vi "PGPASS.ConnectionMgr.vi"(8 "error in (no error)":errorcluster) -> (0 "error out":errorcluster, 3 "Connection":T1)   [LabVIEW 2019, in "PGPASS.lvlib"]
uses:
  PGPASS.lvlib
  PGPASS.Connection Information.ctl
  <vilib>/JDP Science/PostgreSQL Library/Connection/Execute Command (1D string results).vi
  <vilib>/JDP Science/PostgreSQL Library/Connection/Execute Command (Result).vi
  <vilib>/JDP Science/PostgreSQL Library/Result/Get all results as 1D strings array.vi
  <vilib>/JDP Science/PostgreSQL Library/Result/Get Column Headers.vi
  <vilib>/JDP Science/PostgreSQL Library/Result/Clear.vi
  <vilib>/JDP Science/PostgreSQL Library/Connection/PQ Connection.lvclass
panel:
  in  "CANCEL":bool
  out "Status":string
  in  "Validate":bool
  in  "Connections":i32(listbox)
  in  "Exit":bool
  in  "Delete Connection":bool
  in  "Add Connection":bool
  in  "Host":string
  in  "Port":string
  in  "Database":string
  in  "Username":string
  in  "Password":string
  # "PGPASS: Connection Manager"
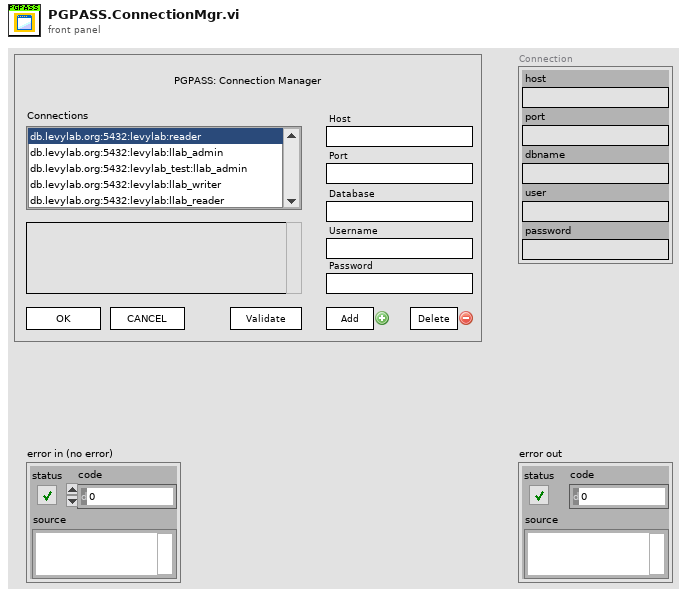
[diagram p1: front panel]
types:
  T1 = typedef "PGPASS.lvlib/PGPASS.Connection Information.ctl" = cluster{"host":string, "port":string, "dbname":string, "user":string, "password":string}
  T2 = enum32{"Invalid", "Standard", "Closed", "Hidden", "Minimized", "Maximized"}
  T3 = enum32{"invalid app kind", "Development System", "Run Time System", "Student Edition", "Embedded LabVIEW", "Evaluation", "Custom"}
  T4 = cluster{"Core":cluster{"Current VI Reference":refnum<vi>, "Close Panel on Exit?":bool}, "All Connections":T1[], "Connection":T1}
  T5 = cluster{"Current VI Reference":refnum<vi>, "Close Panel on Exit?":bool}
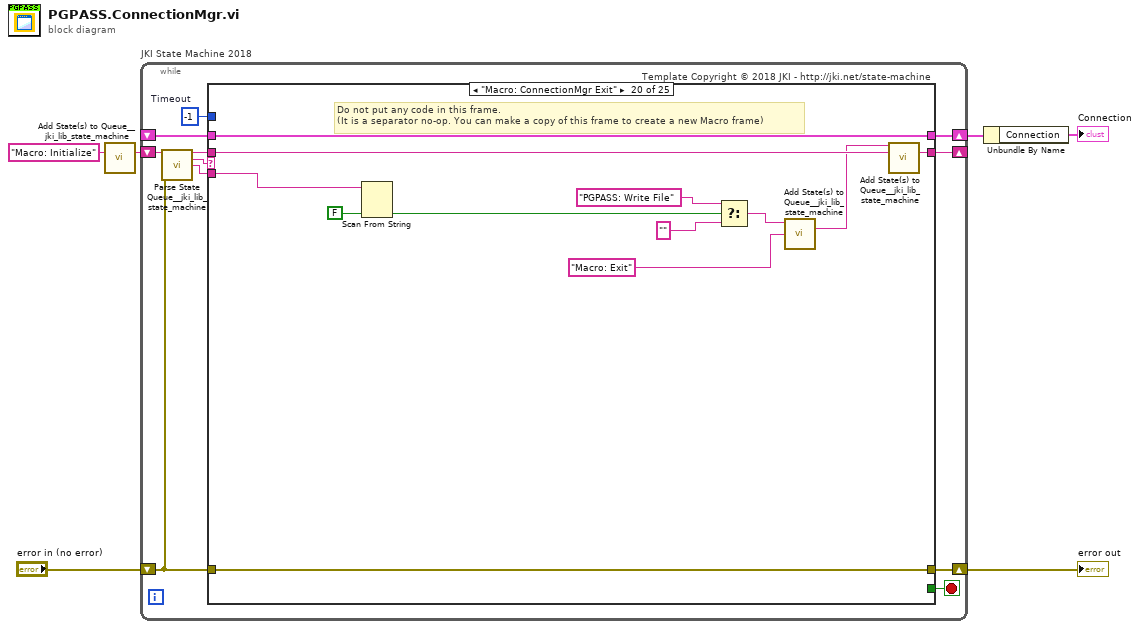
[diagram p0: block diagram]
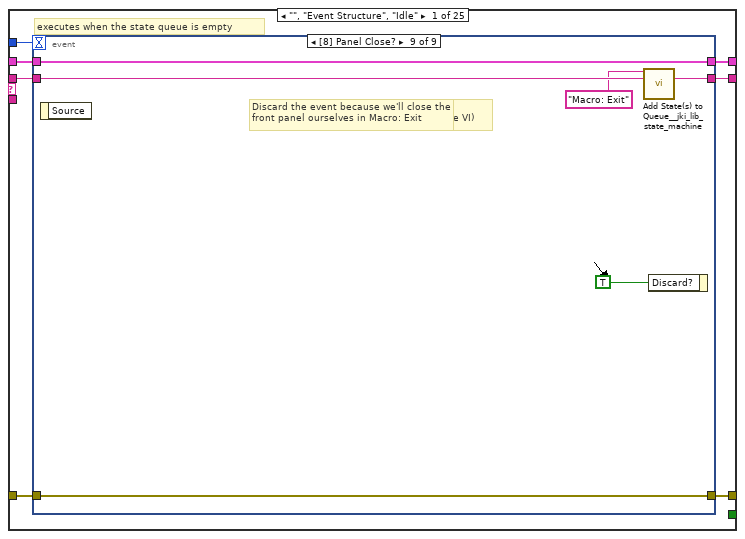
[diagram p2: hidden frame]
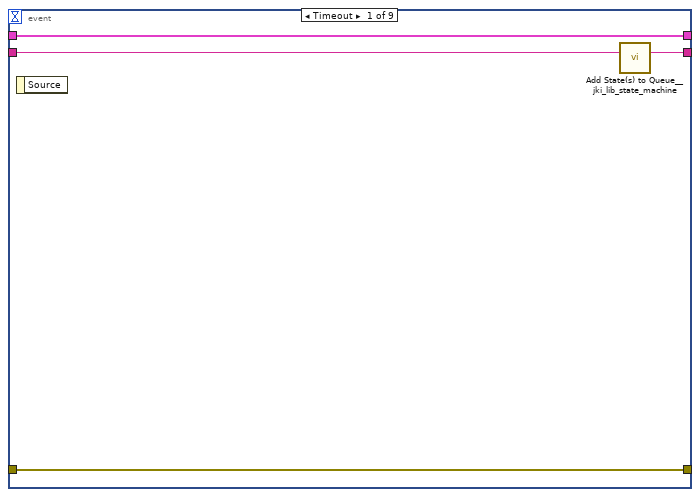
[diagram p3: hidden frame]
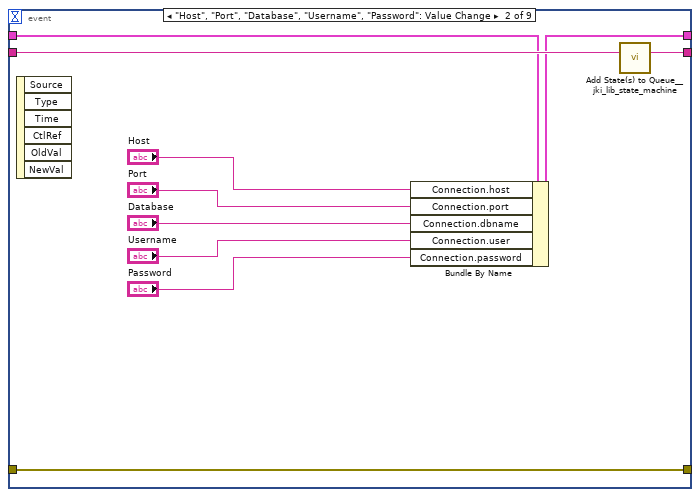
[diagram p4: hidden frame]
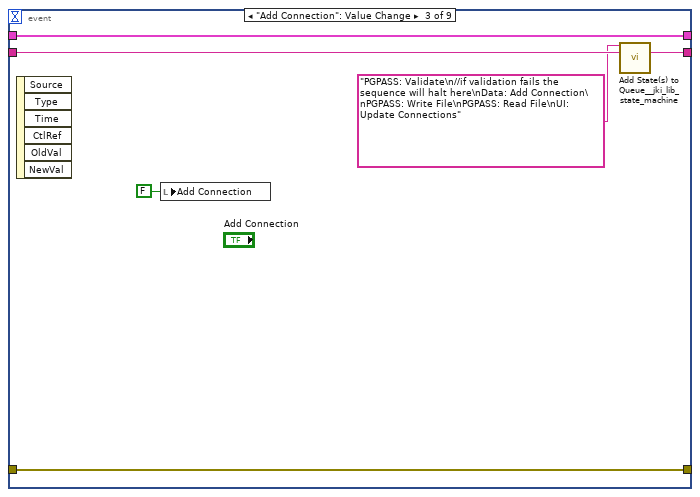
[diagram p5: hidden frame]
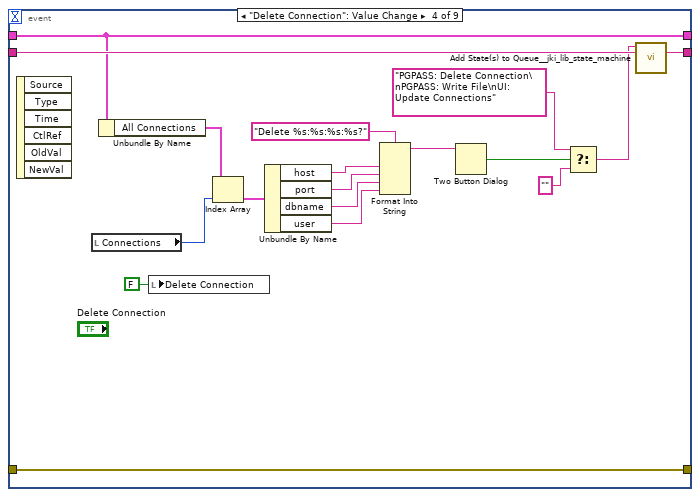
[diagram p6: hidden frame]
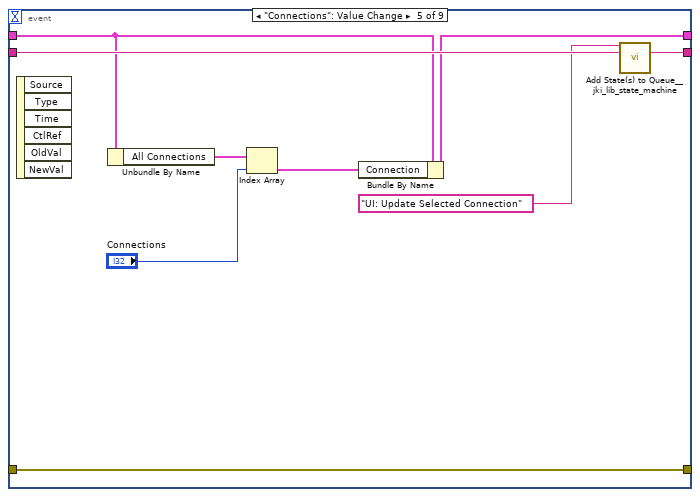
[diagram p7: hidden frame]
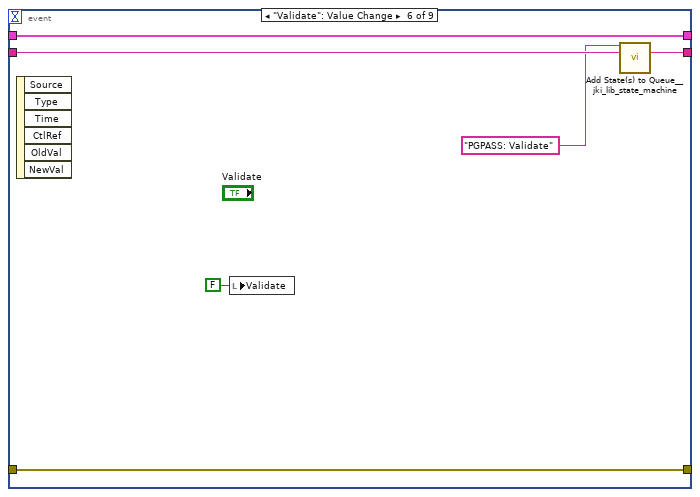
[diagram p8: hidden frame]
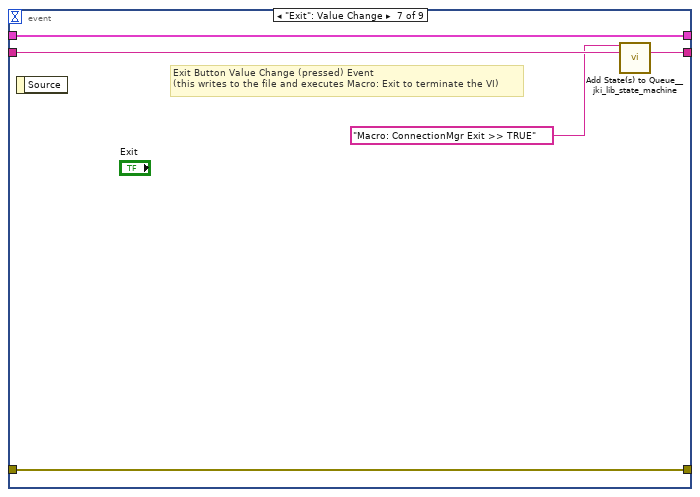
[diagram p9: hidden frame]
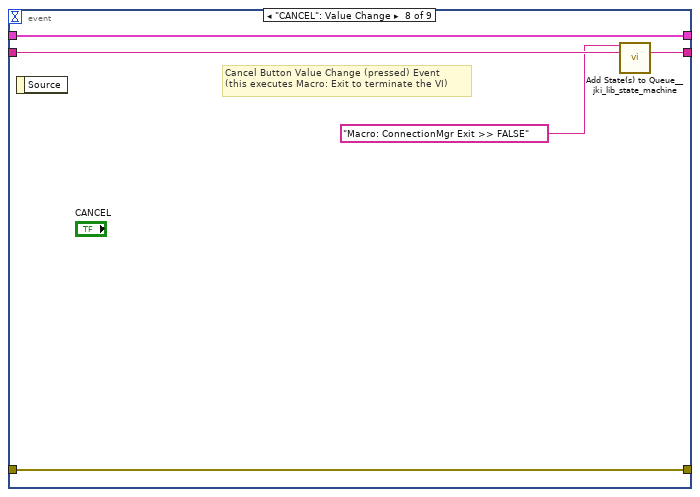
[diagram p10: hidden frame]
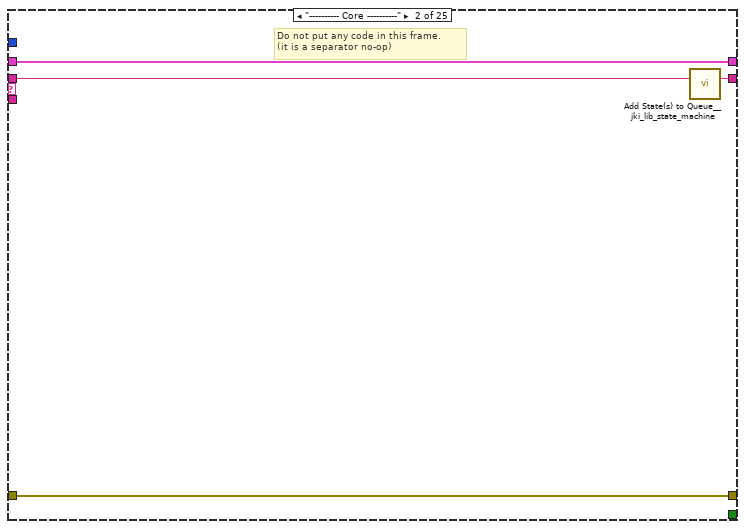
[diagram p11: hidden frame]
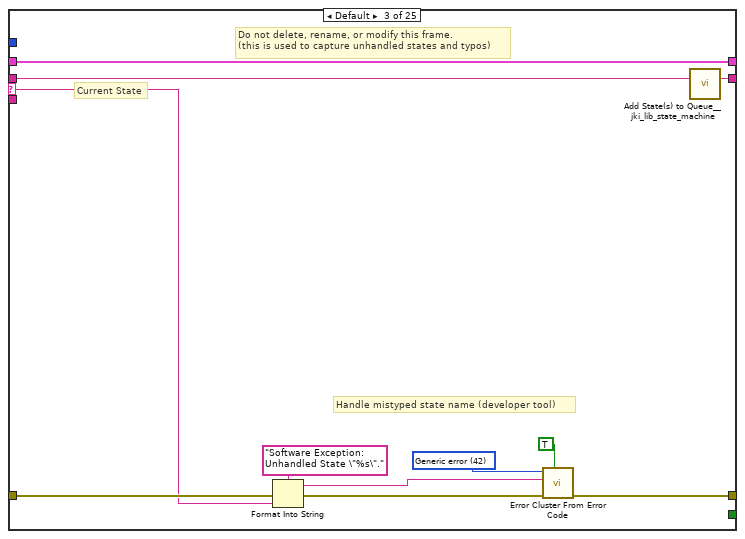
[diagram p12: hidden frame]
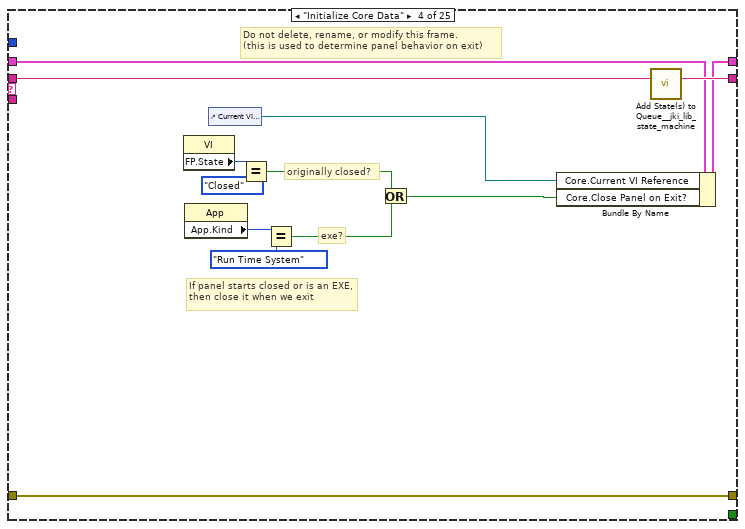
[diagram p13: hidden frame]
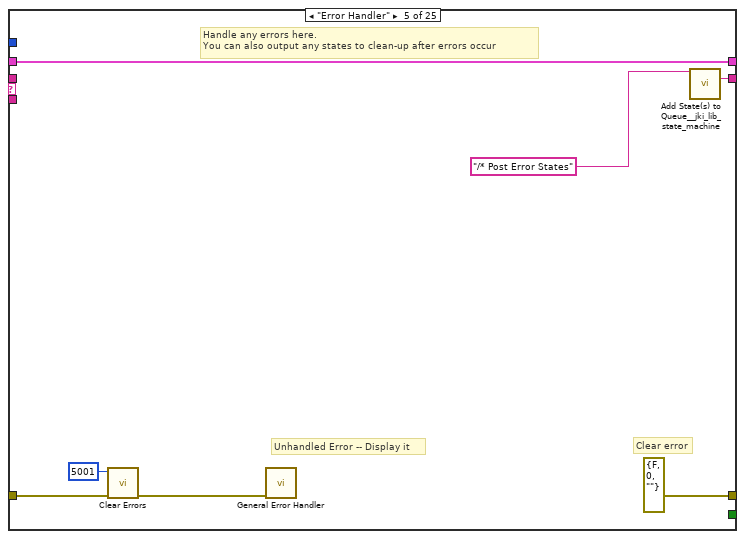
[diagram p14: hidden frame]
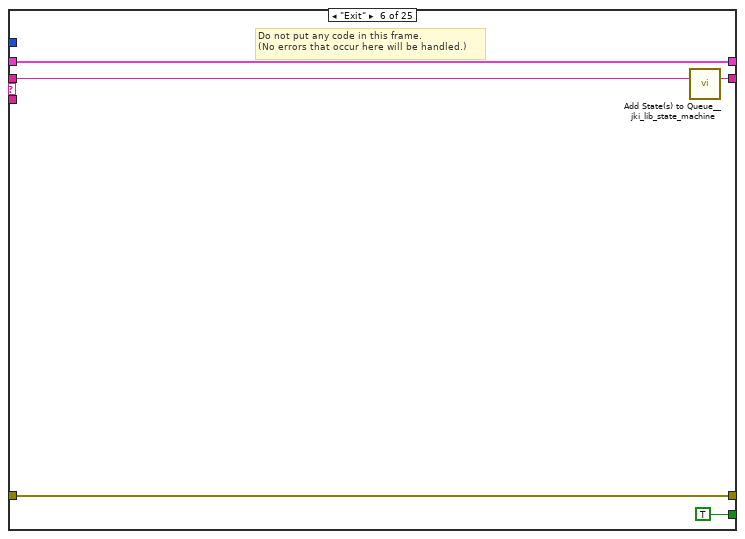
[diagram p15: hidden frame]
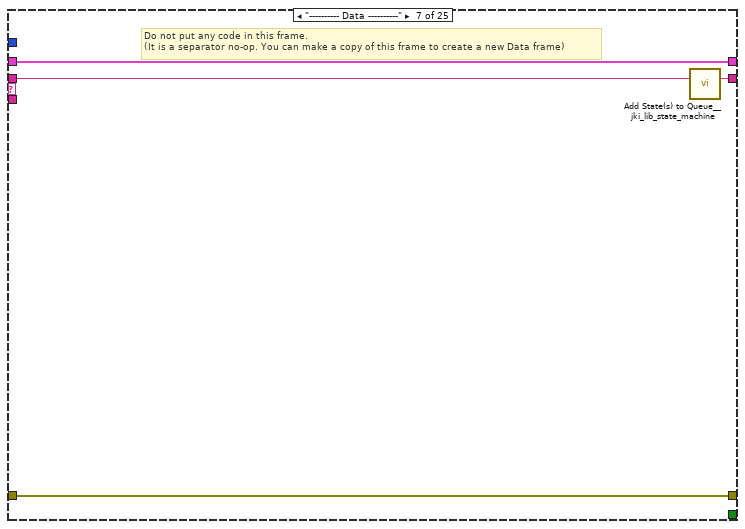
[diagram p16: hidden frame]
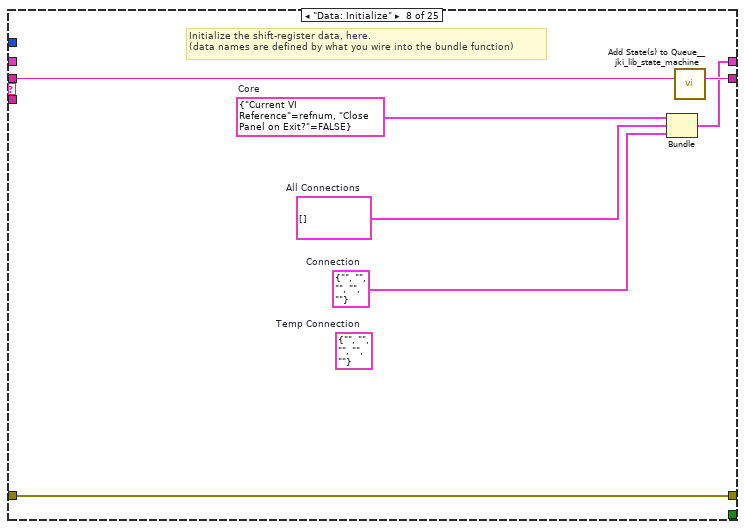
[diagram p17: hidden frame]
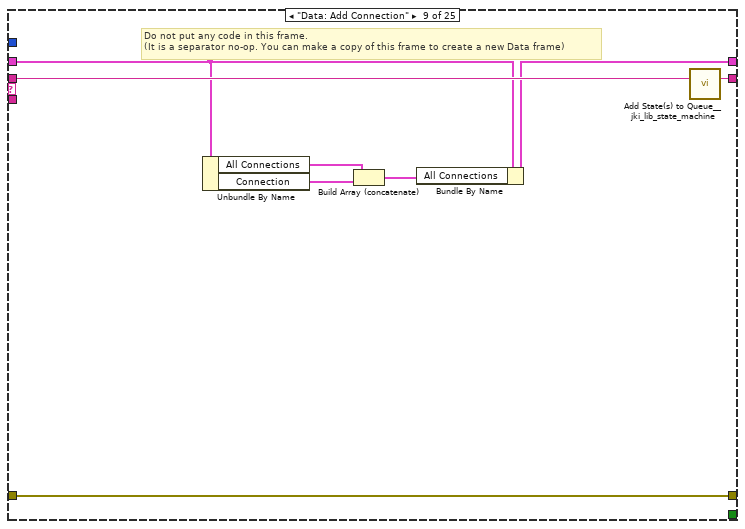
[diagram p18: hidden frame]
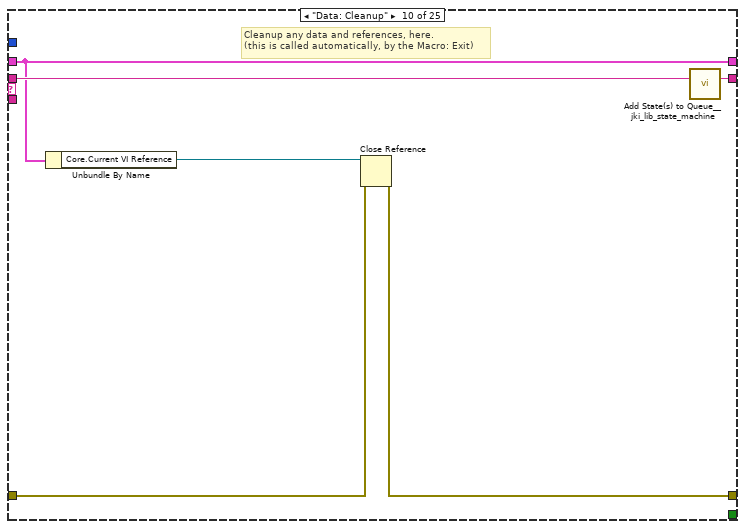
[diagram p19: hidden frame]
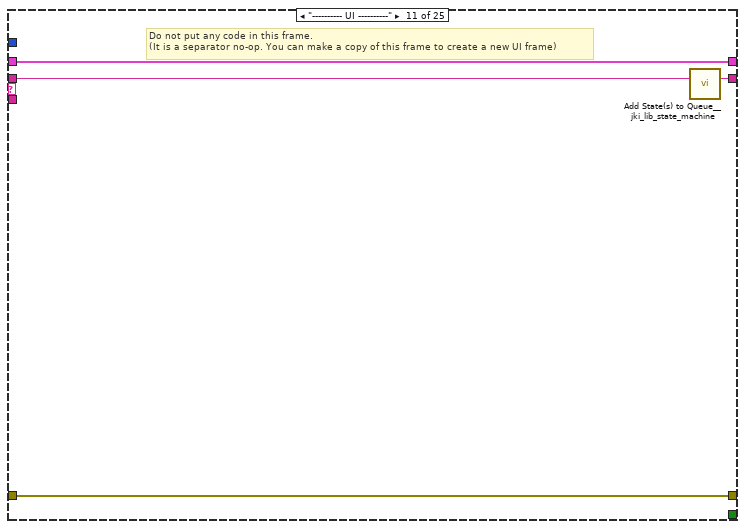
[diagram p20: hidden frame]
diagram:
  n1 = call <vilib>:"Add State(s) to Queue__jki_lib_state_machine.vi"("State(s) in (\"\")"="Macro: Initialize") -> ("States Out"=w6:string)  [unwired: 14 in]
  n2 = while "JKI State Machine 2018" {
    shift-right: [w10] -> w2
    shift-left: _ -> [w9]
    shift-right: [w13] -> w4
    shift-left: "error in (no error)" -> [w7]
    shift-right: [w12] -> _
    shift-left: w6 -> [w14]
    stop <- w11 stop-if-true
    w8 = -1  # Timeout
    # "Template Copyright © 2018 JKI - http://jki.net/state-machine"
    n3 = call <vilib>:"Parse State Queue__jki_lib_state_machine.vi"("State Queue"=w14, "Error In (no error)"=w7) -> ("Remaining States"=w16:string, "Current State"=w17:string, "Arguments"=w15:string)  [unwired: 11 in]
    n4 = case shown="\"Macro: ConnectionMgr Exit\"" w17 {
      selector: w17 -> [_ _ w98 _ _ _ _ _ _ _ _ _ _ _ _ _ _ _ _ _ _ _ _ _ _]
      tunnel: w16 -> [w24 w97 w102 w121 _ w133 w137 w144 w152 w158 w162 w170 w176 w187 w258 w275 w279 w284 w294 w306 w310 w318 w325 w333 w347]
      tunnel: w15 -> [_ _ _ _ _ _ _ _ _ _ _ _ w171 w181 _ _ _ _ _ w297 _ _ _ _ _]
      tunnel: w9 -> [w22 w94 w100 w114 w126 w131 w134 _ w145 w153 w159 w168 w174 w183 w254 w267 w276 w281 w291 w303 w307 w312 w323 w327 w337]
      tunnel: [w21 w95 w104 w118 errorcluster {"status"=FALSE, "code"=0, "source"=""} ("error out") w130 w135 w141 w150 w154 w160 w167 w172 w184 w256 w273 w277 w282 w292 w304 w308 w316 w321 w331 w336] -> w13
      tunnel: w7 -> [w20 w95 w103 w118 w123 w130 w135 w141 w150 w155 w160 w166 w173 w185 w256 w273 w277 w282 w292 w304 w308 w315 w322 w331 w335]
      tunnel: [w23 w96 w101 w120 w128 w132 w136 w143 w151 w157 w161 w169 w175 w186 w257 w274 w278 w283 w293 w305 w309 w317 w324 w332 w346] -> w12
      tunnel: [_ _ _ _ _ TRUE _ _ _ _ _ _ _ _ _ _ _ _ _ _ _ _ _ _ _] -> w11
      tunnel: [w19 w94 w100 w119 w126 w131 w134 w142 w147 w153 w159 w168 w174 w183 w254 w267 w276 w281 w291 w303 w307 w313 w323 w328 w337] -> w10
      tunnel: w8 -> [w18 _ _ _ _ _ _ _ _ _ _ _ _ _ _ _ _ _ _ _ _ _ _ _ _]
      frame "", "Event Structure", "Idle" {
        # "executes when the state queue is empty"
        n5 = event shown="[8] Panel Close?" {
          selector: _ -> [_ _ _ _ _ _ _ _ _]
          dyn-events: _ -> [_ _ _ _ _ _ _ _ _]
          timeout: w18 -> [_ _ _ _ _ _ _ _ _]
          tunnel: w24 -> [w28 w38 w44 w62 w71 w77 w82 w87 w93]
          tunnel: [w27 w37 w43 w61 w70 w76 w81 w86 w92] -> w23
          tunnel: w22 -> [w25 w34 w40 w57 w66 w74 w79 w84 w90]
          tunnel: [w26 w36 w42 w60 w69 w75 w80 w85 w91] -> w21
          tunnel: w20 -> [w26 w36 w42 w60 w69 w75 w80 w85 w91]
          tunnel: [w25 w35 w40 w57 w67 w74 w79 w84 w90] -> w19
          event Timeout {
            n6 = event-data() -> ()  [unwired: 1 in, 1 out]
            n7 = call <vilib>:"Add State(s) to Queue__jki_lib_state_machine.vi"("State(s) in (\"\")"=w28) -> ("States Out"=w27:string)  [unwired: 14 in]
          }
          event "Host", "Port", "Database", "Username", "Password": Value Change {
            n8 = event-data() -> ()  [unwired: 1 in, 6 out]
            n9 = Bundle By Name(cluster=w34, "Connection.host"="Host", "Connection.port"="Port", "Connection.dbname"="Database", "Connection.user"="Username", "Connection.password"="Password") -> (w35:T4)
            n10 = call <vilib>:"Add State(s) to Queue__jki_lib_state_machine.vi"("State(s) in (\"\")"=w38) -> ("States Out"=w37:string)  [unwired: 14 in]
          }
          event "Add Connection": Value Change {
            n11 = event-data() -> ()  [unwired: 1 in, 6 out]
            n12 = local write "Add Connection"(FALSE ("Add Connection")) -> ()
            n13 = call <vilib>:"Add State(s) to Queue__jki_lib_state_machine.vi"("State(s) in Front (\"\")"="PGPASS: Validate\n//if validation fails the sequence will halt here\nData: Add Connection\nPGPASS: Write File\nPGPASS: Read File\nUI: Update Connections" ("State(s) in Front (\"\")"), "State(s) in (\"\")"=w44) -> ("States Out"=w43:string)  [unwired: 13 in]
          }
          event "Delete Connection": Value Change {
            n14 = event-data() -> ()  [unwired: 1 in, 6 out]
            n15 = local read "Connections"() -> (w58:i32)
            n16 = Unbundle By Name(w57) -> ("All Connections"=w59:T1[])
            n17 = local write "Delete Connection"(FALSE ("Delete Connection")) -> ()
            n18 = Index Array(array=w59, index=w58) -> (element=w51:T1)
            n19 = Unbundle By Name(w51) -> ("host"=w55:string, "port"=w54:string, "dbname"=w53:string, "user"=w52:string)
            n20 = Format Into String(format string="Delete %s:%s:%s:%s?", w55, w54, w53, w52) -> (resulting string=w50:string)  [unwired: 2 in, 1 out]
            n21 = Two Button Dialog(message=w50) -> (T button?=w49:bool)  [unwired: 2 in]
            n22 = Select(t="PGPASS: Delete Connection\nPGPASS: Write File\nUI: Update Connections" ("State(s) in Front (\"\")"), s=w49, f="") -> (s? t:f=w48:string)
            n23 = call <vilib>:"Add State(s) to Queue__jki_lib_state_machine.vi"("State(s) in Front (\"\")"=w48, "State(s) in (\"\")"=w62) -> ("States Out"=w61:string)  [unwired: 13 in]
          }
          event "Connections": Value Change {
            n24 = event-data() -> ()  [unwired: 1 in, 6 out]
            n25 = Unbundle By Name(w66) -> ("All Connections"=w68:T1[])
            n26 = Index Array(array=w68, index="Connections") -> (element=w65:T1)
            n27 = Bundle By Name(cluster=w66, "Connection"=w65) -> (w67:T4)
            n28 = call <vilib>:"Add State(s) to Queue__jki_lib_state_machine.vi"("State(s) in Front (\"\")"="UI: Update Selected Connection" ("State(s) in Front (\"\")"), "State(s) in (\"\")"=w71) -> ("States Out"=w70:string)  [unwired: 13 in]
          }
          event "Validate": Value Change {
            n29 = event-data() -> ()  [unwired: 1 in, 6 out]
            n30 = local write "Validate"(FALSE ("Validate")) -> ()
            n31 = call <vilib>:"Add State(s) to Queue__jki_lib_state_machine.vi"("State(s) in Front (\"\")"="PGPASS: Validate" ("State(s) in Front (\"\")"), "State(s) in (\"\")"=w77) -> ("States Out"=w76:string)  [unwired: 13 in]
          }
          event "Exit": Value Change {
            # "Exit Button Value Change (pressed) Event\n(this writes to the file and executes Macro: Exit to terminate the VI)"
            n32 = event-data() -> ()  [unwired: 1 in, 1 out]
            n33 = call <vilib>:"Add State(s) to Queue__jki_lib_state_machine.vi"("State(s) in Front (\"\")"="Macro: ConnectionMgr Exit >> TRUE", "State(s) in (\"\")"=w82) -> ("States Out"=w81:string)  [unwired: 13 in]
          }
          event "CANCEL": Value Change {
            # "Cancel Button Value Change (pressed) Event\n(this executes Macro: Exit to terminate the VI)"
            n34 = event-data() -> ()  [unwired: 1 in, 1 out]
            n35 = call <vilib>:"Add State(s) to Queue__jki_lib_state_machine.vi"("State(s) in Front (\"\")"="Macro: ConnectionMgr Exit >> FALSE", "State(s) in (\"\")"=w87) -> ("States Out"=w86:string)  [unwired: 13 in]
          }
          event Panel Close? {
            # "Discard the event because we'll close the front panel ourselves in Macro: Exit"
            # "Close Panel button (pressed) Event\n(this executes Macro: Exit to terminate the VI)"
            n36 = event-data() -> ()  [unwired: 1 in, 1 out]
            n37 = call <vilib>:"Add State(s) to Queue__jki_lib_state_machine.vi"("State(s) in Front (\"\")"="Macro: Exit", "State(s) in (\"\")"=w93) -> ("States Out"=w92:string)  [unwired: 13 in]
            n38 = event-data("Discard?"=TRUE) -> ()  [unwired: 1 in, 1 out]
          }
        }
      }
      frame "---------- Core ----------" {
        # "Do not put any code in this frame.\n(it is a separator no-op)"
        n39 = call <vilib>:"Add State(s) to Queue__jki_lib_state_machine.vi"("State(s) in (\"\")"=w97) -> ("States Out"=w96:string)  [unwired: 14 in]
      }
      frame Default {
        w107 = 42 items=["No error", "Argument error", "Memory is full", "Out of zone", "End of file", "File already open", "Generic file I/O error", "File not found", "File permission error", "Disk is full", "Duplicate path", "Too many files open", "System feature not enabled", "Resource file not found", "Cannot add resource", "Resource not found", "Image not found", "Image memory error", "Pen does not exist", "Config type invalid", "Config token not found", "Config parse error", "Config memory error", "Bad external code format", "Bad external code offset", "External code not present", "Null window", "Destroy window error", "Null menu", "Print aborted", "Bad print record", "Print driver error", "Windows error during printing", "Memory error during printing", "Print dialog error", "Generic print error", "Invalid device refnum", "Device not found", "Device parameter error", "Device unit error", "Cannot open device", "Device call aborted", "Generic error", "Cancelled by user", "Object ID too low", "Object ID too high", "Object not in heap", "Unknown heap", "Unknown object (invalid DefProc)", "Unknown object (DefProc not in table)", "Message out of range", "Invalid (null) method", "Unknown message", "Manager call not supported", "Bad address", "Network operation in progress", "Network operation timed out", "Connection is busy", "Network attribute not supported", "Network error", "Address in use", "System out of memory", "Connection aborted", "Connection refused", "Not connected", "Already connected", "Connection closed", "Initialization error (interapplication manager)", "Bad occurrence", "Wait on unbound occurrence handler", "Occurrence queue overflow", "Datalog type conflict", "Unused", "Unrecognized type (interapplication manager)", "Memory corrupt", "Failed to make temporary DLL", "Old CIN version", "Drag socket not found", "Failed to load drop-object", "Failed to register OLE object", "Failed to release OLE object", "Format specifier type mismatch", "Unknown format specifier", "Too few format specifiers", "Too many format specifiers", "Scan failed", "Newer CIN version", "Error converting to variant", "Runtime menu error", "Password tampered", "Variant attribute not found", "Incompatible variant data type", "Event data is not available", "Event Store is not present", "Occurrence is not found", "Event Queue is not created", "Event info is not available", "Refnum passed is NULL", "Error retrieving Class GUID", "Error retrieving CoClass GUID", "Error retrieving TypeLib GUID.", "Bad built application magic bytes.", "Specific driver is different from the specific driver associated with the Logical Name.", "There is no session opened to the class driver.", "Max Error", "MAX - Error with config objects", "MAX - Error loading configuration", "MAX - Group not supported"]
        # "Current State"
        # "Do not delete, rename, or modify this frame.\n(this is used to capture unhandled states and typos)"
        # "Handle mistyped state name (developer tool)"
        n40 = Format Into String(format string="Software Exception: Unhandled State \"%s\"." ("message"), error in=w103, w98) -> (resulting string=w106:string, error out=w105:errorcluster)  [unwired: 1 in]
        n41 = call <vilib>:"Error Cluster From Error Code.vi"("show call chain? (False)"=TRUE, "error in (no error)"=w105, "error message (\"\")"=w106, "error code (0)"=w107) -> ("error out"=w104:errorcluster)  [unwired: 5 in]
        n42 = call <vilib>:"Add State(s) to Queue__jki_lib_state_machine.vi"("State(s) in (\"\")"=w102) -> ("States Out"=w101:string)  [unwired: 14 in]
      }
      frame "Initialize Core Data" {
        # "Do not delete, rename, or modify this frame.\n(this is used to determine panel behavior on exit)"
        # "originally closed?"
        # "exe?"
        # "If panel starts closed or is an EXE, then close it when we exit"
        n43 = property class="VI"() -> ("FP.State"=w111:T2)  [unwired: 2 in, 2 out]
        n44 = property class="App"() -> ("App.Kind"=w117:T3)  [unwired: 2 in, 2 out]
        n45 = control-ref of="Current VI Reference"() -> (w112:refnum<vi>)
        n46 = Equal?(x=w111, y=T2."Closed" ("Front Panel Window:State")) -> (x = y?=w109:bool)
        n47 = Equal?(x=w117, y=T3."Run Time System" ("Application:Kind")) -> (x = y?=w115:bool)
        n48 = Or(x=w109, y=w115) -> (x .or. y?=w113:bool)
        n49 = Bundle By Name(cluster=w114, "Core.Current VI Reference"=w112, "Core.Close Panel on Exit?"=w113) -> (w119:T4)
        n50 = call <vilib>:"Add State(s) to Queue__jki_lib_state_machine.vi"("State(s) in (\"\")"=w121) -> ("States Out"=w120:string)  [unwired: 14 in]
      }
      frame "Error Handler" {
        # "Unhandled Error -- Display it"
        # "Handle any errors here.\nYou can also output any states to clean-up after errors occur"
        # "Clear error"
        n51 = call <vilib>:"Clear Errors.vi"("error in (no error)"=w123, "specific error code to clear (0: all)"=5001) -> ("error out"=w124:errorcluster)  [unwired: 4 in, 1 out]
        n52 = call <vilib>:"General Error Handler.vi"("error in (no error)"=w124) -> ()  [unwired: 10 in, 5 out]
        n53 = call <vilib>:"Add State(s) to Queue__jki_lib_state_machine.vi"("State(s) in Front (\"\")"="/* Post Error States") -> ("States Out"=w128:string)  [unwired: 14 in]
      }
      frame "Exit" {
        # "Do not put any code in this frame.\n(No errors that occur here will be handled.)"
        n54 = call <vilib>:"Add State(s) to Queue__jki_lib_state_machine.vi"("State(s) in (\"\")"=w133) -> ("States Out"=w132:string)  [unwired: 14 in]
      }
      frame "---------- Data ----------" {
        # "Do not put any code in this frame.\n(It is a separator no-op. You can make a copy of this frame to create a new Data frame)"
        n55 = call <vilib>:"Add State(s) to Queue__jki_lib_state_machine.vi"("State(s) in (\"\")"=w137) -> ("States Out"=w136:string)  [unwired: 14 in]
      }
      frame "Data: Initialize" {
        (unwired) T1 {"host"="", "port"="", "dbname"="", "user"="", "password"=""}  # Temp Connection
        w138 = T1 {"host"="", "port"="", "dbname"="", "user"="", "password"=""}  # Connection
        w139 = T1[] []  # All Connections
        w140 = T5 {"Current VI Reference"=refnum, "Close Panel on Exit?"=FALSE}  # Core
        # "Initialize the shift-register data, here.\n(data names are defined by what you wire into the bundle function)"
        n56 = Bundle("Core"=w140, "All Connections"=w139, "Connection"=w138) -> (w142:T4)  [unwired: 1 in]
        n57 = call <vilib>:"Add State(s) to Queue__jki_lib_state_machine.vi"("State(s) in (\"\")"=w144) -> ("States Out"=w143:string)  [unwired: 14 in]
      }
      frame "Data: Add Connection" {
        # "Do not put any code in this frame.\n(It is a separator no-op. You can make a copy of this frame to create a new Data frame)"
        n58 = Unbundle By Name(w145) -> ("All Connections"=w149:T1[], "Connection"=w146:T1)
        n59 = Build Array (concatenate)(w149, w146) -> (w148:T1[])
        n60 = Bundle By Name(cluster=w145, "All Connections"=w148) -> (w147:T4)
        n61 = call <vilib>:"Add State(s) to Queue__jki_lib_state_machine.vi"("State(s) in (\"\")"=w152) -> ("States Out"=w151:string)  [unwired: 14 in]
      }
      frame "Data: Cleanup" {
        # "Cleanup any data and references, here.\n(this is called automatically, by the Macro: Exit)"
        n62 = Unbundle By Name(w153) -> ("Core.Current VI Reference"=w156:refnum<vi>)
        n63 = Close Reference(reference=w156, error in (no error)=w155) -> (error out=w154:errorcluster)
        n64 = call <vilib>:"Add State(s) to Queue__jki_lib_state_machine.vi"("State(s) in (\"\")"=w158) -> ("States Out"=w157:string)  [unwired: 14 in]
      }
      frame "---------- UI ----------" {
        # "Do not put any code in this frame.\n(It is a separator no-op. You can make a copy of this frame to create a new UI frame)"
        n65 = call <vilib>:"Add State(s) to Queue__jki_lib_state_machine.vi"("State(s) in (\"\")"=w162) -> ("States Out"=w161:string)  [unwired: 14 in]
      }
      frame "UI: Initialize" {
        # "Initialize the User Interface, here.\n(this is called automatically, by the Macro: Init)"
        n66 = local write "Status"("" ("Status")) -> ()
        n67 = call <userlib>:"Fit VI window to Largest Dec__ogtk.vi"("error in (no error)"=w166, "border spacing (2 px)"=0) -> ("error out"=w167:errorcluster)  [unwired: 4 in, 1 out]
        n68 = property on="Connections" class="LstBox (strict)"("Val(Sgnl)"=0 ("Value (Signaling)")) -> ()  [unwired: 2 in, 2 out]
        n69 = call <vilib>:"Add State(s) to Queue__jki_lib_state_machine.vi"("State(s) in (\"\")"=w170) -> ("States Out"=w169:string)  [unwired: 14 in]
      }
      frame "UI: Cursor Set" {
        # "Argument"
        # "Set and Unset Cursor Busy.\n(Usage: \"UI: Cursor Set >> Busy|Idle\")"
        n70 = case shown="\"Idle\", Default" w171 {
          tunnel: w173 -> [w178 w180]
          tunnel: [w177 w179] -> w172
          frame "Idle", Default {
            n71 = call <vilib>:"Unset Busy.vi"("error in (no error)"=w178) -> ("error out"=w177:errorcluster)  [unwired: 10 in]
          }
          frame "Busy" {
            n72 = call <vilib>:"Set Busy.vi"("error in (no error)"=w180) -> ("error out"=w179:errorcluster)  [unwired: 9 in, 1 out]
          }
        }
        n73 = call <vilib>:"Add State(s) to Queue__jki_lib_state_machine.vi"("State(s) in (\"\")"=w176) -> ("States Out"=w175:string)  [unwired: 14 in]
      }
      frame "UI: Front Panel State" {
        # "Argument"
        # "Set Front Panel Open or Closed\n(Usage: \"UI: Front Panel State >> Open|Close\")"
        n74 = Unbundle By Name(w183) -> ("Core.Current VI Reference"=w182:refnum<vi>)
        n75 = case shown="\"Minimize\", \"Minimized\"" w181 {
          tunnel: w185 -> [w193 w208 w219 w232 w245]
          tunnel: [w195 w209 w221 w234 w247] -> w184
          tunnel: w182 -> [w194 w206 w220 w233 w246]
          frame "Open", "Standard", Default {
            w188 = T2."Standard" ("State")
            n76 = property class="VI"(reference=w194, error in=w193) -> (reference out=w191:refnum<vi>, error out=w192:errorcluster, "FP.State"=w190:T2)
            n77 = Not Equal?(x=w190, y=w188) -> (x != y?=w189:bool)
            n78 = case shown="True" w189 {
              tunnel: [w199 w201] -> w195
              tunnel: w192 -> [w198 w201]
              tunnel: w191 -> [w197 _]
              tunnel: w188 -> [w196 _]
              frame True {
                n79 = invoke class="VI" method="FP.Open"(reference=w197, error in=w198, "Activate"=TRUE, "State"=w196) -> (error out=w199:errorcluster)  [unwired: 1 in, 4 out]
              }
              frame False {
              }
            }
          }
          frame "Close", "Closed" {
            n80 = property class="VI"(reference=w206, error in=w208) -> (reference out=w205:refnum<vi>, error out=w207:errorcluster, "FP.State"=w203:T2)
            n81 = Not Equal?(x=w203, y=T2."Closed" ("Front Panel Window:State")) -> (x != y?=w202:bool)
            n82 = case shown="True" w202 {
              tunnel: [w210 w213] -> w209
              tunnel: w207 -> [w210 w212]
              tunnel: w205 -> [_ w211]
              frame False {
              }
              frame True {
                n83 = invoke class="VI" method="FP.Close"(reference=w211, error in=w212) -> (error out=w213:errorcluster)  [unwired: 1 in, 2 out]
              }
            }
          }
          frame "Hidden", "Hide" {
            w214 = T2."Hidden" ("State")
            n84 = property class="VI"(reference=w220, error in=w219) -> (reference out=w217:refnum<vi>, error out=w218:errorcluster, "FP.State"=w216:T2)
            n85 = Not Equal?(x=w216, y=w214) -> (x != y?=w215:bool)
            n86 = case shown="True" w215 {
              tunnel: [w225 w226] -> w221
              tunnel: w218 -> [w224 w226]
              tunnel: w217 -> [w223 _]
              tunnel: w214 -> [w222 _]
              frame True {
                n87 = invoke class="VI" method="FP.Open"(reference=w223, error in=w224, "State"=w222) -> (error out=w225:errorcluster)  [unwired: 2 in, 4 out]
              }
              frame False {
              }
            }
          }
          frame "Minimize", "Minimized" {
            w227 = T2."Minimized" ("State")
            n88 = property class="VI"(reference=w233, error in=w232) -> (reference out=w230:refnum<vi>, error out=w231:errorcluster, "FP.State"=w229:T2)
            n89 = Not Equal?(x=w229, y=w227) -> (x != y?=w228:bool)
            n90 = case shown="True" w228 {
              tunnel: [w238 w239] -> w234
              tunnel: w231 -> [w237 w239]
              tunnel: w230 -> [w236 _]
              tunnel: w227 -> [w235 _]
              frame True {
                n91 = invoke class="VI" method="FP.Open"(reference=w236, error in=w237, "State"=w235) -> (error out=w238:errorcluster)  [unwired: 2 in, 4 out]
              }
              frame False {
              }
            }
          }
          frame "Maximize", "Maximized" {
            w240 = T2."Maximized" ("State")
            n92 = property class="VI"(reference=w246, error in=w245) -> (reference out=w243:refnum<vi>, error out=w244:errorcluster, "FP.State"=w242:T2)
            n93 = Not Equal?(x=w242, y=w240) -> (x != y?=w241:bool)
            n94 = case shown="True" w241 {
              tunnel: [w251 w252] -> w247
              tunnel: w244 -> [w250 w252]
              tunnel: w243 -> [w249 _]
              tunnel: w240 -> [w248 _]
              frame True {
                n95 = invoke class="VI" method="FP.Open"(reference=w249, error in=w250, "State"=w248) -> (error out=w251:errorcluster)  [unwired: 2 in, 4 out]
              }
              frame False {
              }
            }
          }
        }
        n96 = call <vilib>:"Add State(s) to Queue__jki_lib_state_machine.vi"("State(s) in (\"\")"=w187) -> ("States Out"=w186:string)  [unwired: 14 in]
      }
      frame "UI: Update Connections" {
        # "Do not put any code in this frame.\n(It is a separator no-op. You can make a copy of this frame to create a new UI frame)"
        n97 = Unbundle By Name(w254) -> ("All Connections"=w253:T1[])
        n98 = for {
          tunnel: w253 -> [w265] mode=indexing
          tunnel: [w259] -> w255 mode=indexing
          n99 = Unbundle By Name(w265) -> ("host"=w263:string, "port"=w262:string, "dbname"=w261:string, "user"=w260:string)
          n100 = Format Into String(format string="%s:%s:%s:%s", w263, w262, w261, w260) -> (resulting string=w259:string)  [unwired: 2 in, 1 out]
        }
        n101 = property on="Connections" class="LstBox (strict)"("Item Names"=w255) -> ()  [unwired: 2 in, 2 out]
        n102 = call <vilib>:"Add State(s) to Queue__jki_lib_state_machine.vi"("State(s) in (\"\")"=w258) -> ("States Out"=w257:string)  [unwired: 14 in]
      }
      frame "UI: Update Selected Connection" {
        (unwired) "" ("password")
        # "Do not put any code in this frame.\n(It is a separator no-op. You can make a copy of this frame to create a new UI frame)"
        n103 = Unbundle By Name(w267) -> ("Connection"=w266:T1)
        n104 = Unbundle By Name(w266) -> ("host"=w270:string, "port"=w271:string, "dbname"=w272:string, "user"=w269:string, "password"=w268:string)
        n105 = local write "Port"(w271) -> ()
        n106 = local write "Username"(w269) -> ()
        n107 = local write "Password"(w268) -> ()
        n108 = local write "Database"(w272) -> ()
        n109 = local write "Host"(w270) -> ()
        n110 = call <vilib>:"Add State(s) to Queue__jki_lib_state_machine.vi"("State(s) in (\"\")"=w275) -> ("States Out"=w274:string)  [unwired: 14 in]
      }
      frame "---------- Macro ----------" {
        # "Do not put any code in this frame.\n(It is a separator no-op. You can make a copy of this frame to create a new Macro frame)"
        n111 = call <vilib>:"Add State(s) to Queue__jki_lib_state_machine.vi"("State(s) in (\"\")"=w279) -> ("States Out"=w278:string)  [unwired: 14 in]
      }
      frame "Macro: Initialize" {
        w280 = "Data: Initialize\nInitialize Core Data\nUI: Initialize\nUI: Front Panel State >> Open\n\nPGPASS: Read File\nUI: Update Connections"  # Data: Initialize Initialize Core Data UI: Initialize UI: Front Panel State >> Open  PGPASS: Read File UI: Update Connections
        # "Initialization Macro\n(This is called once, when the VI starts)"
        n112 = call <vilib>:"Add State(s) to Queue__jki_lib_state_machine.vi"("State(s) in Front (\"\")"=w280, "State(s) in (\"\")"=w284) -> ("States Out"=w283:string)  [unwired: 13 in]
      }
      frame "Macro: Exit" {
        # "Exit Macro\n(This is called once, when the VI exits)"
        n113 = Unbundle By Name(w291) -> ("Core.Close Panel on Exit?"=w290:bool)
        n114 = Select(t="UI: Front Panel State >> Close", s=w290, f="") -> (s? t:f=w287:string)
        n115 = call <vilib>:"Add State(s) to Queue__jki_lib_state_machine.vi"("State(s) in (\"\")"=w287, "State(s) at Back (\"\")"="Data: Cleanup\nExit") -> ("States Out"=w285:string)  [unwired: 13 in]
        n116 = call <vilib>:"Add State(s) to Queue__jki_lib_state_machine.vi"("State(s) in Front (\"\")"=w285, "State(s) in (\"\")"=w294) -> ("States Out"=w293:string)  [unwired: 13 in]
      }
      frame "Macro: ConnectionMgr Exit" {
        # "Do not put any code in this frame.\n(It is a separator no-op. You can make a copy of this frame to create a new Macro frame)"
        n117 = Scan From String(input string=w297, default 1=FALSE) -> (output 1=w295:bool)  [unwired: 3 in, 3 out]
        n118 = Select(t="PGPASS: Write File", s=w295, f="") -> (s? t:f=w301:string)
        n119 = call <vilib>:"Add State(s) to Queue__jki_lib_state_machine.vi"("State(s) in Front (\"\")"=w301, "State(s) at Back (\"\")"="Macro: Exit") -> ("States Out"=w299:string)  [unwired: 13 in]
        n120 = call <vilib>:"Add State(s) to Queue__jki_lib_state_machine.vi"("State(s) in Front (\"\")"=w299, "State(s) in (\"\")"=w306) -> ("States Out"=w305:string)  [unwired: 13 in]
      }
      frame "---------- PGPASS ----------" {
        # "Template Separator\n(You can make a copy of, or modify, this frame)"
        n121 = call <vilib>:"Add State(s) to Queue__jki_lib_state_machine.vi"("State(s) in (\"\")"=w310) -> ("States Out"=w309:string)  [unwired: 14 in]
      }
      frame "PGPASS: Read File" {
        # "Read PGPASS file\n(and populate Connections array)"
        n122 = call "PGPASS.Read.vi"("error in"=w315) -> ("error out"=w316:errorcluster, "Connections"=w314:T1[])  [unwired: 9 in]
        n123 = Bundle By Name(cluster=w312, "All Connections"=w314) -> (w313:T4)
        n124 = call <vilib>:"Add State(s) to Queue__jki_lib_state_machine.vi"("State(s) in Front (\"\")"="" ("State(s) in Front (\"\")"), "State(s) in (\"\")"=w318) -> ("States Out"=w317:string)  [unwired: 13 in]
      }
      frame "PGPASS: Write File" {
        # "Read PGPASS file\n(and populate Connections array)"
        n125 = Unbundle By Name(w323) -> ("All Connections"=w320:T1[])
        n126 = call "PGPASS.Write.vi"("error in"=w322, "Connections"=w320) -> ("error out"=w321:errorcluster)  [unwired: 9 in]
        n127 = call <vilib>:"Add State(s) to Queue__jki_lib_state_machine.vi"("State(s) in Front (\"\")"="" ("State(s) in Front (\"\")"), "State(s) in (\"\")"=w325) -> ("States Out"=w324:string)  [unwired: 13 in]
      }
      frame "PGPASS: Delete Connection" {
        # "Template Separator\n(You can make a copy of, or modify, this frame)"
        n128 = Unbundle By Name(w327) -> ("All Connections"=w330:T1[])
        n129 = local read "Connections"() -> (w329:i32)
        n130 = Delete From Array(array=w330, index=w329) -> (array with subset deleted=w326:T1[])  [unwired: 1 in, 1 out]
        n131 = Bundle By Name(cluster=w327, "All Connections"=w326) -> (w328:T4)
        n132 = call <vilib>:"Add State(s) to Queue__jki_lib_state_machine.vi"("State(s) in (\"\")"=w333) -> ("States Out"=w332:string)  [unwired: 14 in]
      }
      frame "PGPASS: Validate" {
        # "Validate Selected Connection\n(and populate Connections array)"
        n133 = Unbundle By Name(w337) -> ("Connection"=w340:T1)
        n134 = local write "Status"("" ("Status")) -> ()
        n135 = call "PGPASS.Format Connection String with Password.vi"("error in"=w335, "Connection Information"=w340) -> ("error out"=w338:errorcluster, "connection string"=w339:string)  [unwired: 8 in]
        n136 = call <vilib>:"Connect.vi"("error in (no error)"=w338, "Connection Strings"=w339) -> ("error out"=w344:errorcluster, "PQ Connection"=w345:refnum<class "PQ Connection.lvclass">)  [unwired: 8 in]
        n137 = case shown="No Error" w344 {
          selector: w344 -> [w352 w357]
          tunnel: w345 -> [w356 w358]
          tunnel: [w348 w359] -> w343
          tunnel: [w351 w357] -> w342
          tunnel: [w350 w358] -> w341
          frame No Error {
            n138 = call-poly <vilib>:"Execute.vi"("error in (no error)"=w352, "SQL"="SELECT version();", "PQ Connection in"=w356) -> ("error out"=w351:errorcluster, "Result (Rows or Columns)"=w353:string[], "PQ Connection out"=w350:refnum<class "PQ Connection.lvclass">)  [unwired: 4 in, 2 out]
            n139 = Index Array(array=w353) -> (element=w349:string)  [unwired: 1 in]
            n140 = Format Into String(format string="Connection OK:\n%s", w349) -> (resulting string=w348:string)  [unwired: 2 in, 1 out]
          }
          frame Error {
            n141 = Unbundle By Name(w357) -> ("source"=w360:string)
            n142 = Format Into String(format string="Connection Bad:\n%s", w360) -> (resulting string=w359:string)  [unwired: 2 in, 1 out]
          }
        }
        "Status" <- w343
        n143 = call <vilib>:"Disconnect.vi"("error in (no error)"=w342, "PQ Connection in"=w341) -> ("error out"=w336:errorcluster)  [unwired: 9 in]
        n144 = call <vilib>:"Add State(s) to Queue__jki_lib_state_machine.vi"("State(s) in (\"\")"=w347) -> ("States Out"=w346:string)  [unwired: 14 in]
      }
    }
  }
  "error out" <- w4
  n145 = Unbundle By Name(w2) -> ("Connection"=→"Connection":T1)
